vi "Reset.vi"(8 "error in (no error)":errorcluster caption="entrée d'erreur (pas d'erreur)", 11 "Class Shielding_ Box JC-PB3044 en entrée":refnum<class "Class Shielding_ Box JC-PB3044.lvclass">) -> (0 "error out":errorcluster caption="sortie d'erreur", 3 "Class Shielding_ Box JC-PB3044 en sortie":refnum<class "Class Shielding_ Box JC-PB3044.lvclass">)   [LabVIEW 2020, in "Library Instrument & Equipement.lvlib" / "Library Shielding box.lvlib" / "Class Shielding_ Box JC-PB3044.lvclass"]
uses:
  Class Shielding_ Box JC-PB3044.lvclass
  C:/Users/ngarcin/OneDrive - Altyor/Standard TB/Class/Shielding box/Class Shielding box (Default)/Class Shielding_ Box (Default).lvclass
  Class Shielding_ Box JC-PB3044.lvclass/Class Shielding_ Box JC-PB3044.ctl
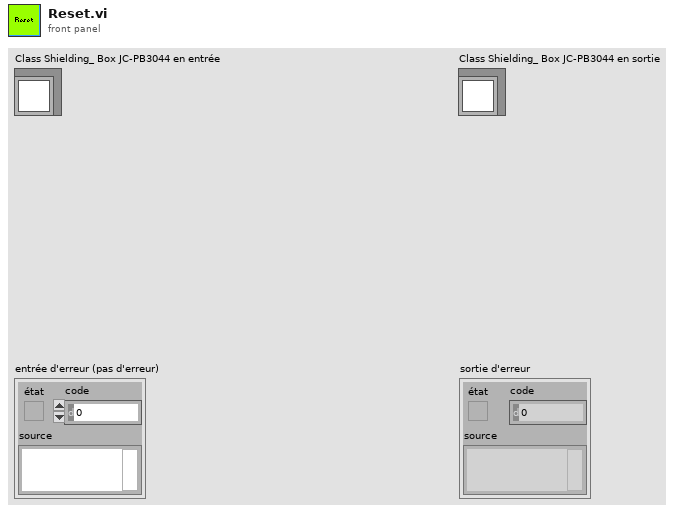
[diagram p1: front panel]
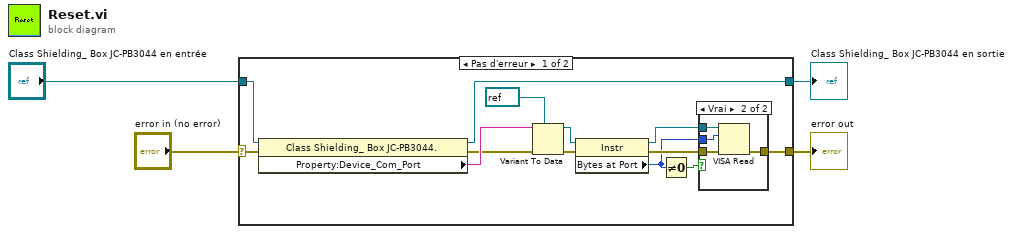
[diagram p0: block diagram]
diagram:
  n1 = case shown="Pas d'erreur" "error in (no error)" {
    selector: "error in (no error)" -> [w10 w24]
    tunnel: [w16 w24] -> w1
    tunnel: [w11 w23] -> w3
    tunnel: "Class Shielding_ Box JC-PB3044 en entrée" -> [w17 w23]
    frame No Error {
      n2 = property class="Class Shielding_ Box JC-PB3044."(reference=w17, error in=w10) -> (reference out=w11:refnum<class "Class Shielding_ Box JC-PB3044.lvclass">, error out=w6:errorcluster, "Property:Device_Com_Port"=w9:string)
      n3 = Variant To Data(error in=w6, type=refnum<visa-resource-name> refnum ("référence en sortie"), Variant=w9) -> (data=w7:refnum<visa-resource-name>, error out=w5:errorcluster)
      n4 = property class="Instr"(reference=w7, error in=w5) -> (reference out=w14:refnum<visa-resource-name>, error out=w15:errorcluster, "Bytes at Port"=w13:u32)
      n5 = Not Equal To 0?(x=w13) -> (x != 0?=w12:bool)
      n6 = case shown="Vrai" w12 {
        tunnel: [w18 w22] -> w16
        tunnel: w13 -> [_ w21]
        tunnel: w15 -> [w18 w20]
        tunnel: w14 -> [_ w19]
        frame False {
        }
        frame True {
          n7 = VISA Read(VISA resource name=w19, byte count=w21, error in (no error)=w20) -> (error out=w22:errorcluster)  [unwired: 3 out]
        }
      }
    }
    frame Error {
    }
  }
  "error out" <- w1
  "Class Shielding_ Box JC-PB3044 en sortie" <- w3
